vi "获取采集硬件的测量值练习.vi"() -> ()   [LabVIEW 2025]
uses:
  <vilib>/Instr/_visa.llb/VISA Configure Serial Port (Instr).vi
panel:
  out "地址01的光亮度数据":u64
  out "转换为十进制数据":u32
  out "字符串显示·的十六进制数据":string
  out "无符号字节数组":u8[](array[numeric])
  out "十六进制整形字符串":string[](array[string])
  out "提取的从机地址01的亮度原始数据":string
  out "获取下位机返回的原始数据包":string
  in  "发送命令":string
  in  "波特率":u32=9600 caption="波特率(9600)"
  in  "选择串口":refnum<visa-resource-name>
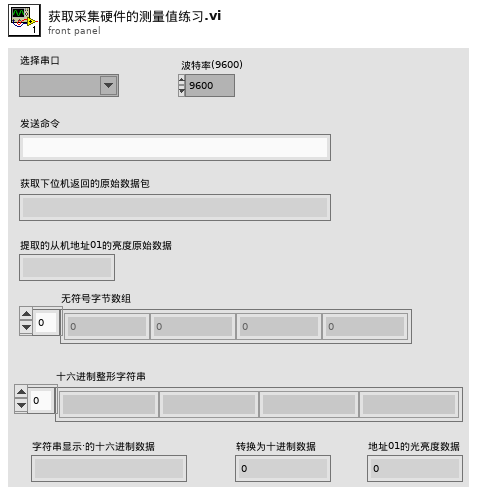
[diagram p1: front panel]
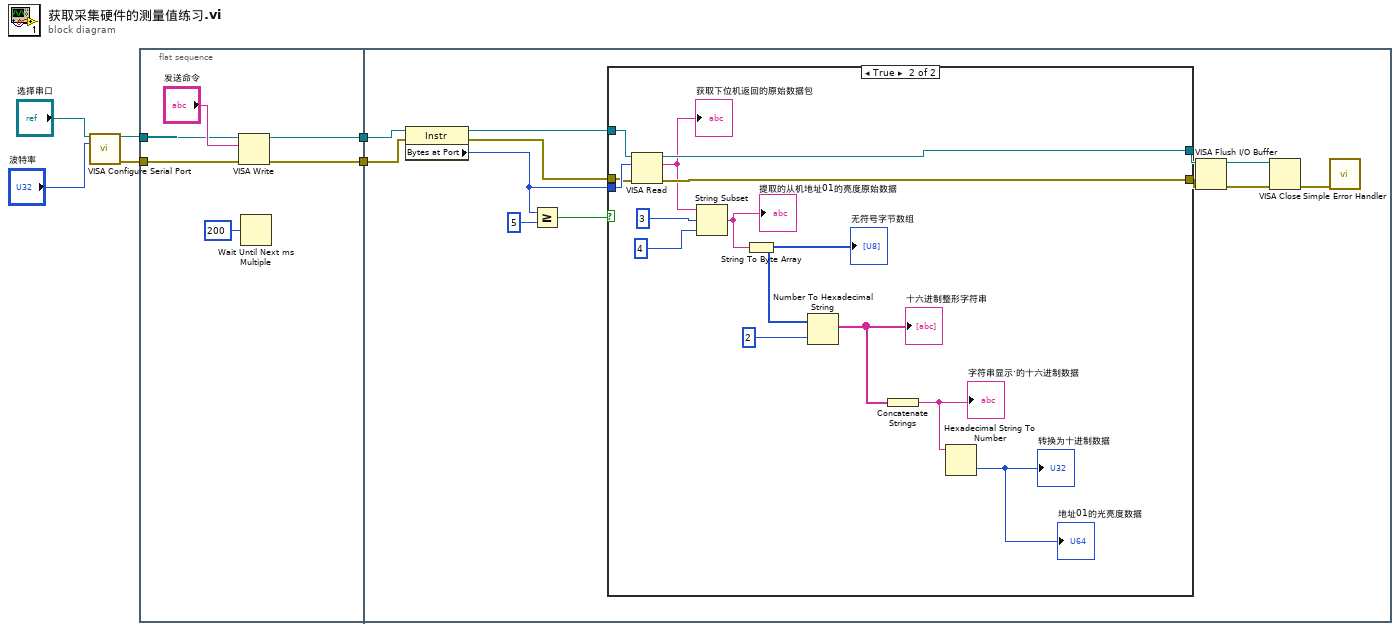
[diagram p0: block diagram]
diagram:
  n1 = call-poly "VISA Configure Serial Port"("VISA resource name"="选择串口", "baud rate (9600)"="波特率") -> ("VISA resource name out"=w4:refnum<visa-resource-name>, "error out"=w3:errorcluster)  [unwired: 12 in]
  n2 = flat-sequence {
    tunnel: w4 -> [w11]
    tunnel: w3 -> [w10]
    tunnel: [w8] -> w2
    tunnel: [w7] -> w1
    tunnel: w2 -> [w24]
    tunnel: w1 -> [w23]
    frame #0 {
      n3 = VISA Write(VISA resource name=w11, write buffer="发送命令", error in (no error)=w10) -> (VISA resource name out=w8:refnum<visa-resource-name>, error out=w7:errorcluster)  [unwired: 1 out]
      n4 = Wait Until Next ms Multiple(millisecond multiple=u32 200 ("毫秒倍数")) -> ()  [unwired: 1 out]
    }
    frame #1 {
      n5 = property class="Instr"(reference=w24, error in=w23) -> (reference out=w20:refnum<visa-resource-name>, error out=w18:errorcluster, "Bytes at Port"=w19:u32)
      n6 = Greater Or Equal?(x=w19, y=u32 5) -> (x >= y?=w22:bool)
      n7 = case shown="True" w22 {
        tunnel: w20 -> [w26 w40]
        tunnel: w19 -> [_ w39]
        tunnel: w18 -> [w25 w38]
        tunnel: [w26 w33] -> w14
        tunnel: [w25 w32] -> w13
        frame False {
        }
        frame True {
          n8 = VISA Read(VISA resource name=w40, byte count=w39, error in (no error)=w38) -> (VISA resource name out=w33:refnum<visa-resource-name>, read buffer=w31:string, error out=w32:errorcluster)  [unwired: 1 out]
          "获取下位机返回的原始数据包" <- w31
          n9 = String Subset(string=w31, offset (0)=3 ("偏移量(0)"), length (rest)=4 ("长度（剩余）")) -> (substring=w35:string)
          "提取的从机地址01的亮度原始数据" <- w35
          n10 = String To Byte Array(string=w35) -> (unsigned byte array=w30:u8[])
          "无符号字节数组" <- w30
          n11 = Number To Hexadecimal String(1:i16 2 ("宽度(-)"), 2:w30) -> (0:w29:string[])
          "十六进制整形字符串" <- w29
          n12 = Concatenate Strings(w29) -> (w28:string)
          "字符串显示·的十六进制数据" <- w28
          n13 = Hexadecimal String To Number(string=w28) -> (number=→"地址01的光亮度数据" →"转换为十进制数据":u32)  [unwired: 2 in, 1 out]
        }
      }
      n14 = VISA Flush I/O Buffer(VISA resource name=w14, error in (no error)=w13) -> (VISA resource name out=w15:refnum<visa-resource-name>, error out=w16:errorcluster)  [unwired: 1 in]
      n15 = VISA Close(VISA resource name=w15, error in (no error)=w16) -> (error out=w17:errorcluster)
      n16 = call <vilib>:"Simple Error Handler.vi"("error in (no error)"=w17) -> ()  [unwired: 4 in, 5 out]
    }
  }
